vi "AcionaEletrovalvula2.vi"(11 "queue Variaveis":refnum<queue>) -> ()   [LabVIEW 2019]
panel:
  in  "Stop":bool
  in  "Frequência":dbl
  in  "Duty Cycle %":dbl=50.0 min=0.0 max=100.0 step=1.0
  in  "Valvula in":bool=TRUE
  in  "Automático":bool
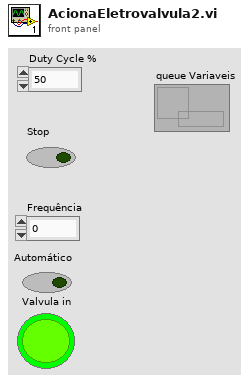
[diagram p1: front panel]
types:
  T1 = cluster{"Automatico":bool, "Valvula":bool, "Duty cycle":dbl, "Stop":bool, "Frequencia":dbl}
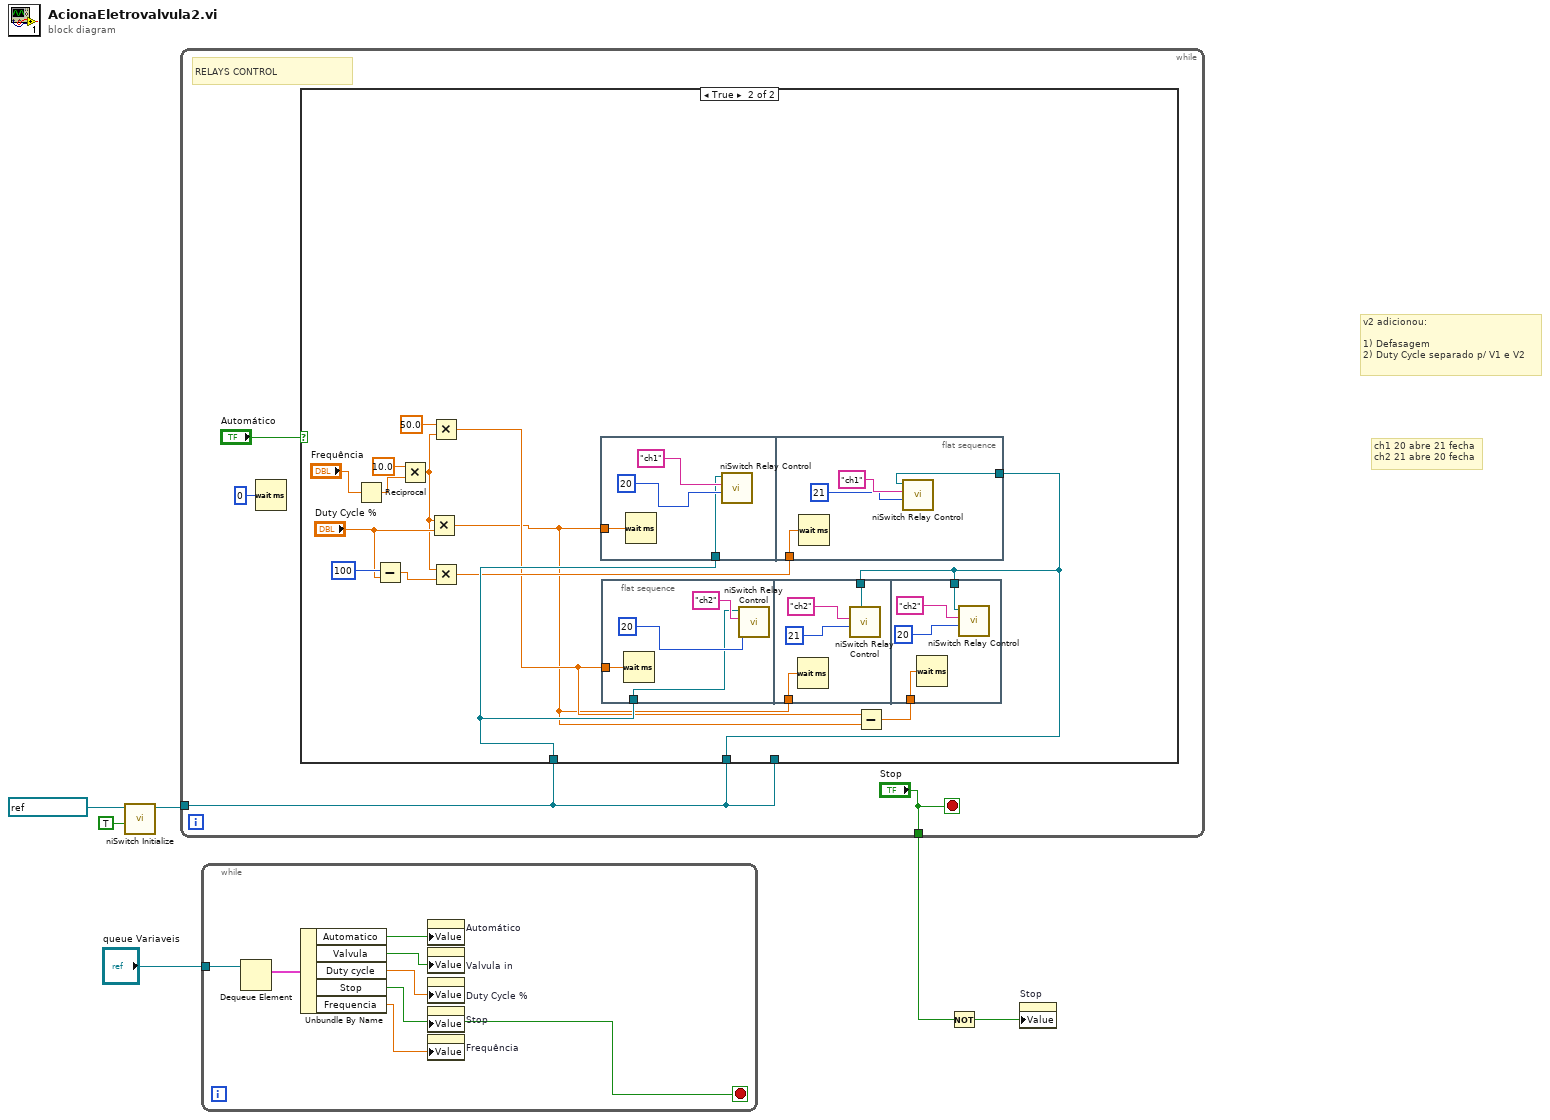
[diagram p0: block diagram]
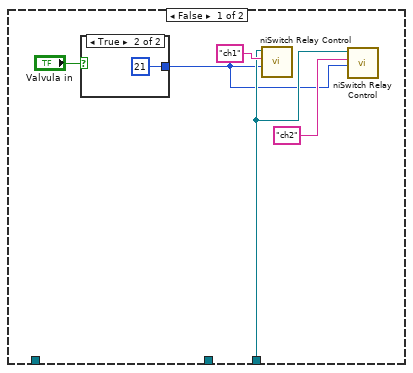
[diagram p2: hidden frame]
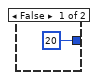
[diagram p3: hidden frame]
diagram:
  # "ch1 20 abre 21 fecha\nch2 21 abre 20 fecha"
  # "v2 adicionou:\n\n1) Defasagem\n2) Duty Cycle separado p/ V1 e V2"
  n1 = call <instrlib>:"niSwitch Initialize.vi"("reset device (boolean value)"=TRUE, "resource name"=refnum<k15> "SC1Mod3") -> ("instrument handle out"=w6:refnum<k15>)  [unwired: 8 in, 1 out]
  n2 = while {
    tunnel: w6 -> [w8]
    tunnel: ["Stop"] -> w3
    stop <- "Stop" stop-if-true
    # "RELAYS CONTROL"
    n3 = Wait (ms)(milliseconds to wait=u32 0) -> ()  [unwired: 1 out]
    n4 = case shown="True" "Automático" {
      tunnel: w8 -> [w12 _]
      tunnel: w8 -> [_ w25]
      tunnel: w8 -> [_ w21]
      frame False {
        n5 = case shown="True" "Valvula in" {
          tunnel: [20 21] -> w11
          frame False {
          }
          frame True {
          }
        }
        n6 = call <instrlib>:"niSwitch Relay Control.vi"("relay action (Close Relay)"=w11, "relay names"="ch1" ("String"), "instrument handle"=w12) -> ()  [unwired: 7 in, 2 out]
        n7 = call <instrlib>:"niSwitch Relay Control.vi"("relay action (Close Relay)"=w11, "relay names"="ch2" ("String"), "instrument handle"=w12) -> ()  [unwired: 7 in, 2 out]
      }
      frame True {
        n8 = Reciprocal(x="Frequência") -> (1/x=w31:dbl)
        n9 = Subtract(x=100, y="Duty Cycle %") -> (x-y=w27:dbl)
        n10 = Multiply(x=10.0 ("y"), y=w31) -> (x*y=w22:dbl)
        n11 = Multiply(x=w22, y="Duty Cycle %") -> (x*y=w19:dbl)
        n12 = Multiply(x=50.0, y=w22) -> (x*y=w20:dbl)
        n13 = Multiply(x=w22, y=w27) -> (x*y=w24:dbl)
        n14 = flat-sequence {
          tunnel: w25 -> [w33]
          tunnel: w19 -> [w32]
          tunnel: w21 -> [w37]
          tunnel: w24 -> [w36]
          frame #0 {
            n15 = Wait (ms)(milliseconds to wait=w32) -> ()  [unwired: 1 out]
            n16 = call <instrlib>:"niSwitch Relay Control.vi"("relay action (Close Relay)"=20, "relay names"="ch1" ("String"), "instrument handle"=w33) -> ()  [unwired: 7 in, 2 out]
          }
          frame #1 {
            n17 = Wait (ms)(milliseconds to wait=w36) -> ()  [unwired: 1 out]
            n18 = call <instrlib>:"niSwitch Relay Control.vi"("relay action (Close Relay)"=21, "relay names"="ch1" ("String"), "instrument handle"=w37) -> ()  [unwired: 7 in, 2 out]
          }
        }
        n19 = flat-sequence {
          tunnel: w25 -> [w41]
          tunnel: w20 -> [w40]
          tunnel: w21 -> [w45]
          tunnel: w19 -> [w44]
          tunnel: w21 -> [w49]
          tunnel: w18 -> [w48]
          frame #0 {
            n20 = Wait (ms)(milliseconds to wait=w40) -> ()  [unwired: 1 out]
            n21 = call <instrlib>:"niSwitch Relay Control.vi"("relay action (Close Relay)"=20, "relay names"="ch2" ("String"), "instrument handle"=w41) -> ()  [unwired: 7 in, 2 out]
          }
          frame #1 {
            n22 = Wait (ms)(milliseconds to wait=w44) -> ()  [unwired: 1 out]
            n23 = call <instrlib>:"niSwitch Relay Control.vi"("relay action (Close Relay)"=21, "relay names"="ch2" ("String"), "instrument handle"=w45) -> ()  [unwired: 7 in, 2 out]
          }
          frame #2 {
            n24 = Wait (ms)(milliseconds to wait=w48) -> ()  [unwired: 1 out]
            n25 = call <instrlib>:"niSwitch Relay Control.vi"("relay action (Close Relay)"=20, "relay names"="ch2" ("String"), "instrument handle"=w49) -> ()  [unwired: 7 in, 2 out]
          }
        }
        n26 = Subtract(x=w20, y=w19) -> (x-y=w18:dbl)
      }
    }
  }
  n27 = while {
    tunnel: "queue Variaveis" -> [w58]
    stop <- w52 stop-if-true
    n28 = Dequeue Element(queue=w58) -> (element=w57:T1)  [unwired: 2 in, 3 out]
    n29 = Unbundle By Name(w57) -> ("Automatico"=w56:bool, "Valvula"=w55:bool, "Duty cycle"=w54:dbl, "Stop"=w52:bool, "Frequencia"=w53:dbl)
    n30 = property on="Automático" class="Bool (strict)"("Value"=w56) -> ()  [unwired: 2 in, 2 out]
    n31 = property on="Valvula in" class="Bool (strict)"("Value"=w55) -> ()  [unwired: 2 in, 2 out]
    n32 = property on="Duty Cycle %" class="DigNum (strict)"("Value"=w54) -> ()  [unwired: 2 in, 2 out]
    n33 = property on="Stop" class="Bool (strict)"("Value"=w52) -> ()  [unwired: 2 in, 2 out]
    n34 = property on="Frequência" class="DigNum (strict)"("Value"=w53) -> ()  [unwired: 2 in, 2 out]
  }
  n35 = Not(x=w3) -> (.not. x?=w2:bool)
  n36 = property on="Stop" class="Bool (strict)"("Value"=w2) -> ()  [unwired: 2 in, 2 out]
